vi "TEST Set Wind Speeds.vi"() -> ()   [LabVIEW 2011]
doc: "This is is part of the test process for the Wind Turbine SEQ class. It works in conjunction with the TEST Get Wind Speeds.vi\n\nAAL 9/09"
panel:
  in  "Exit":bool
  in  "Set Speed":bool
  in  "Turbine":u16(ring) items=["Wind Turbine #1", "Wind Turbine #2", "Wind Turbine #3"]
  in  "Wind Speed (m/s)":dbl
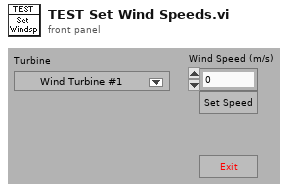
[diagram p1: front panel]
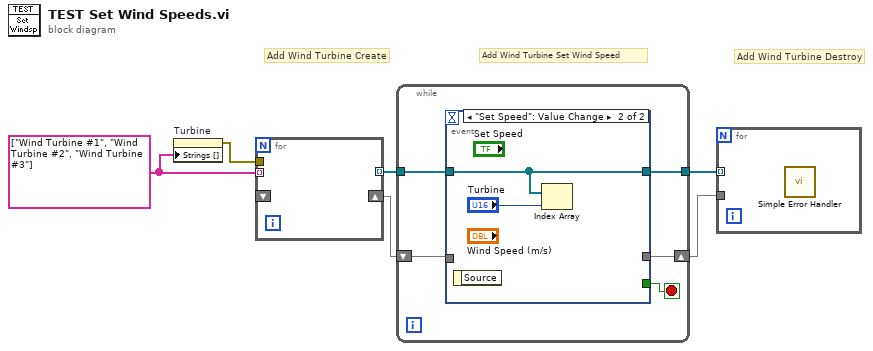
[diagram p0: block diagram]
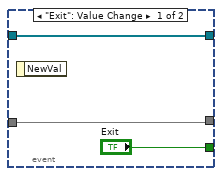
[diagram p2: hidden frame]
diagram:
  w6 = string[] ["Wind Turbine #1", "Wind Turbine #2", "Wind Turbine #3"]
  # "Add Wind Turbine Destroy"
  # "Add Wind Turbine Set Wind Speed"
  # "Add Wind Turbine Create"
  n1 = property on="Turbine" class="Ring (strict)"("Strings []"=w6) -> (error out=w3:errorcluster)  [unwired: 2 in, 1 out]
  n2 = for {
    tunnel: w6 -> [w10] mode=indexing
    tunnel: [w9] -> w5 mode=indexing
    tunnel: w3 -> [_]
    shift-right: [w8] -> w2
    shift-left: _ -> [w7]
  }
  n3 = while {
    tunnel: w5 -> [w14]
    tunnel: [w13] -> w4
    shift-right: [w12] -> w1
    shift-left: w2 -> [w11]
    stop <- w15 stop-if-true
    n4 = event shown="[1] \"Set Speed\": Value Change" {
      selector: _ -> [_ _]
      dyn-events: _ -> [_ _]
      timeout: _ -> [_ _]
      tunnel: ["Exit" _] -> w15
      tunnel: w14 -> [w17 w21]
      tunnel: [w17 w21] -> w13
      tunnel: w11 -> [w16 w19]
      tunnel: [w16 _] -> w12
      event "Exit": Value Change {
        n5 = event-data() -> ()  [unwired: 2 out]
      }
      event "Set Speed": Value Change {
        n6 = event-data() -> ()  [unwired: 2 out]
        n7 = Index Array(array=w21, index="Turbine") -> ()  [unwired: 1 out]
      }
    }
  }
  n8 = for {
    tunnel: w4 -> [_] mode=indexing
    tunnel: w1 -> [_]
    n9 = call <vilib>:"Simple Error Handler.vi"() -> ()  [unwired: 2 in, 8 out]
  }
